vi "Get Phase.vi"(8 "error in (no error)":errorcluster, 11 "RP Instrument in":refnum<class "RP Instrument.lvclass">) -> (0 "error out":errorcluster, 2 "Phase":u32=1 format="0x%x (%d)", 3 "RP Instrument out":refnum<class "RP Instrument.lvclass">)   [LabVIEW 2019, in "RP Instrument.lvclass"]
uses:
  RP Instrument.lvclass
  RP Status Offsets.ctl
  RP Instrument.lvclass/RP Instrument.ctl
  RP Communicator/RP Communicator.lvclass
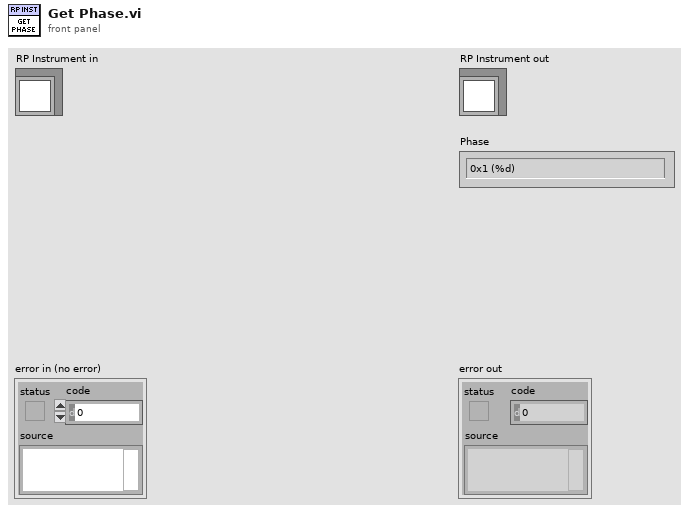
[diagram p1: front panel]
types:
  T1 = typedef "RP Status Offsets.ctl" = u16
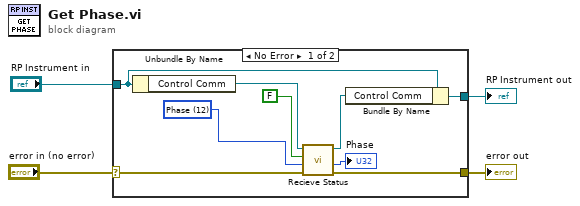
[diagram p0: block diagram]
diagram:
  n1 = case shown="No Error" "error in (no error)" {
    selector: "error in (no error)" -> [w10 w15]
    tunnel: [w9 w15] -> w3
    tunnel: [w6 w14] -> w1
    tunnel: "RP Instrument in" -> [w7 w14]
    frame No Error {
      w5 = T1 12 items=["Writer address"=0, "Record start position"=4, "Trig state etc."=8, "Phase"=12, "RxFIFO counter"=24, "TxFIFO counter"=28] ("Status offset")
      n2 = Unbundle By Name(w7) -> ("Control Comm"=w13:refnum<class "RP Communicator.lvclass">)
      n3 = call-dynamic "Recieve Status.vi"("error in (no error)"=w10, "Status offset"=w5, "Read config instead"=FALSE, "RP Communicator in"=w13) -> ("error out"=w9:errorcluster, "Status response"=→"Phase":u32, "RP Communicator out"=w12:refnum<class "RP Communicator.lvclass">)  [unwired: 5 in]
      n4 = Bundle By Name(cluster=w7, "Control Comm"=w12) -> (w6:refnum<class "RP Instrument.lvclass">)
    }
    frame Error {
    }
  }
  "error out" <- w3
  "RP Instrument out" <- w1
